vi "Get New Level.vi"(8 "error in (no error)":cluster{"状态":bool, "代码":i32, "源":string} caption="错误输入（无错误）", 11 "水位输入":refnum<class "Water Level.lvclass">) -> (0 "error out":cluster{"状态":bool, "代码":i32, "源":string} caption="错误输出", 2 "水位":dbl, 3 "水位输出":refnum<class "Water Level.lvclass">)   [LabVIEW 2013, in "Water Level.lvlib" / "Water Level.lvclass"]
doc: "子类绝不可对该VI进行重写。如需对子类添加任何功能，应对Get Water Level.vi进行重写。"
uses:
  Water Level.lvclass
  <vilib>/ActorFramework/Actor/Actor.lvclass/Actor.ctl
  Water Level.lvclass/Water Level.ctl
  Update Water Level Msg/Update Water Level Msg.lvclass
  <vilib>/ActorFramework/Actor/Actor.lvclass
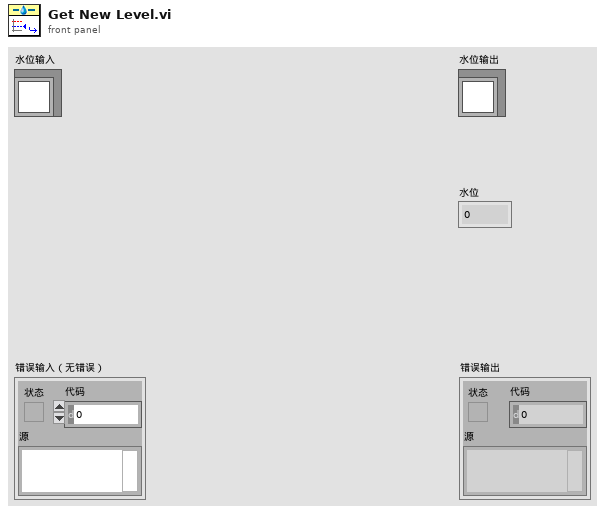
[diagram p1: front panel]
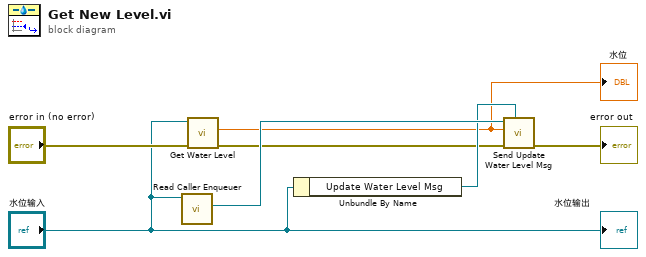
[diagram p0: block diagram]
diagram:
  n1 = call <vilib>:"Read Caller Enqueuer.vi"("Actor"="水位输入") -> ("Caller Enqueuer"=w6:refnum<class "Message Enqueuer.lvclass">)  [unwired: 10 in]
  n2 = call-dynamic "Get Water Level.vi"("error in (no error)"="error in (no error)", "水位输入"="水位输入") -> ("error out"=w4:cluster{"状态":bool, "代码":i32, "源":string}, "水位"=w1:dbl)  [unwired: 8 in]
  "水位" <- w1
  n3 = Unbundle By Name("水位输入") -> ("Update Water Level Msg"=w5:refnum<class "Update Water Level Msg.lvclass">)
  n4 = call "Send Update Water Level Msg.vi"("更新水位消息"=w5, "error in (no error)"=w4, "水位"=w1, "消息待入队列"=w6) -> ("error out"=→"error out":cluster{"状态":bool, "代码":i32, "源":string})  [unwired: 7 in]
  "水位输出" <- "水位输入"
